vi "Unknown Command.vi"(8 "error in (no error)":errorcluster, 10 "String":string, 11 "Process In":refnum<class "Process.lvclass">) -> (0 "error out":errorcluster, 3 "Process Out":refnum<class "Process.lvclass">)   [LabVIEW 2020, in "Process.lvclass"]
uses:
  Process.lvclass
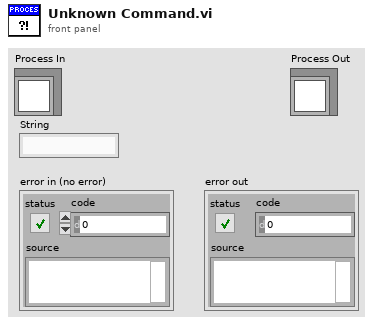
[diagram p1: front panel]
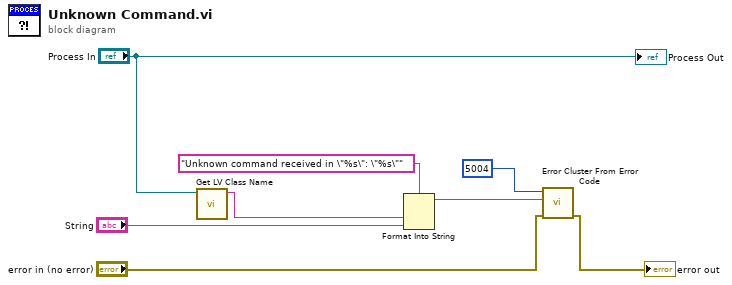
[diagram p0: block diagram]
diagram:
  n1 = call <vilib>:"Get LV Class Name.vi"("object"="Process In") -> ("class name"=w1:string)  [unwired: 9 in, 1 out]
  n2 = Format Into String(format string="Unknown command received in \"%s\": \"%s\"", w1, "String") -> (resulting string=w8:string)  [unwired: 2 in, 1 out]
  n3 = call <vilib>:"Error Cluster From Error Code.vi"("error in (no error)"="error in (no error)", "error message (\"\")"=w8, "error code (0)"=5004) -> ("error out"=→"error out":errorcluster)  [unwired: 6 in]
  "Process Out" <- "Process In"
